vi "Untitled 2 (SubVI).vi"(11 "Digital in":refnum<vi>) -> ()   [LabVIEW 2020]
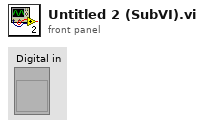
[diagram p1: front panel]
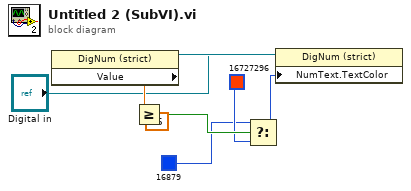
[diagram p0: block diagram]
diagram:
  n1 = property class="DigNum (strict)"(reference="Digital in") -> (reference out=w4:refnum<vi>, "Value"=w3:dbl)  [unwired: 1 in, 1 out]
  n2 = Greater Or Equal?(x=w3, y=0.5) -> (x >= y?=w7:bool)
  n3 = Select(t=u32 16879 ("Numeric Text.Text Colors:Text Color"), s=w7, f=u32 16727296 ("Numeric Text.Text Colors:Text Color")) -> (s? t:f=w8:u32)
  n4 = property class="DigNum (strict)"(reference=w4, "NumText.TextColor"=w8) -> ()  [unwired: 1 in, 2 out]
